vi "HTML Index Save.vi"(8 "error in (no error)":errorcluster, 10 "title":string) -> (0 "error out":errorcluster)   [LabVIEW 2014, in "lvprj2html.lvlib"]
uses:
  lvprj2html.lvlib
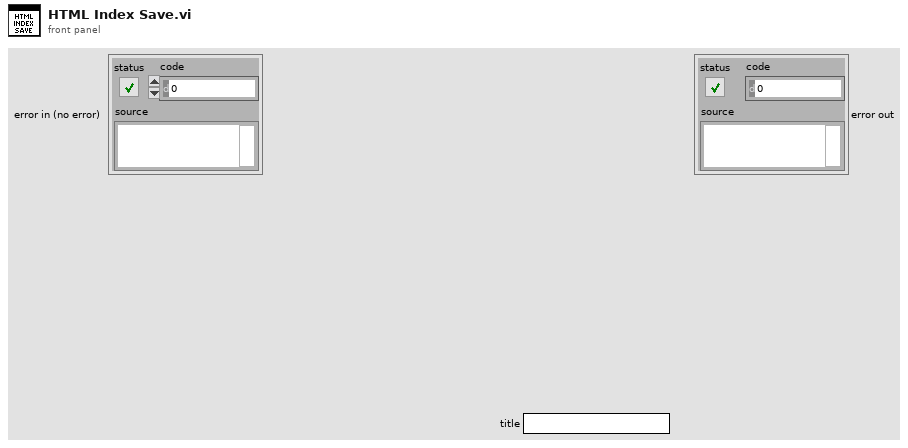
[diagram p1: front panel]
types:
  T1 = enum16{"open", "replace", "create", "open or create", "replace or create", "replace or create with confirmation"}
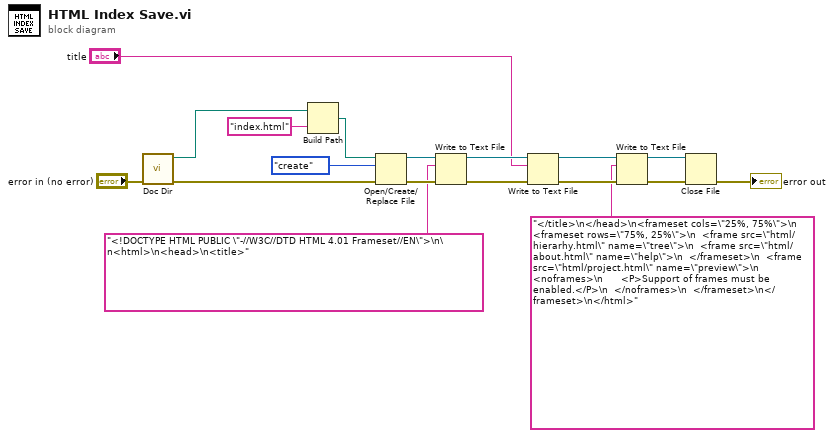
[diagram p0: block diagram]
diagram:
  n1 = call "Doc Dir.vi"("error in (no error)"="error in (no error)") -> ("error out"=w11:errorcluster, "appended path"=w12:path)  [unwired: 9 in]
  n2 = Build Path(base path=w12, name or relative path="index.html") -> (appended path=w16:path)
  n3 = Open/Create/Replace File(file path (use dialog)=w16, error in=w11, operation (0:open)=T1."create") -> (refnum out=w18:refnum<file>, error out=w14:errorcluster)  [unwired: 3 in, 1 out]
  n4 = Write to Text File(file (use dialog)=w18, text="<!DOCTYPE HTML PUBLIC \"-//W3C//DTD HTML 4.01 Frameset//EN\">\n\n<html>\n<head>\n<title>", error in=w14) -> (refnum out=w7:refnum<file>, error out=w4:errorcluster)  [unwired: 1 in, 1 out]
  n5 = Write to Text File(file (use dialog)=w7, text="title", error in=w4) -> (refnum out=w6:refnum<file>, error out=w5:errorcluster)  [unwired: 1 in, 1 out]
  n6 = Write to Text File(file (use dialog)=w6, text="</title>\n</head>\n<frameset cols=\"25%, 75%\">\n  <frameset rows=\"75%, 25%\">\n  <frame src=\"html/hierarhy.html\" name=\"tree\">\n  <frame src=\"html/about.html\" name=\"help\">\n  </frameset>\n  <frame src=\"html/project.html\" name=\"preview\">\n  <noframes>\n      <P>Support of frames must be enabled.</P>\n  </noframes>\n  </frameset>\n</frameset>\n</html>", error in=w5) -> (refnum out=w9:refnum<file>, error out=w10:errorcluster)  [unwired: 1 in, 1 out]
  n7 = Close File(refnum=w9, error in=w10) -> (error out=→"error out":errorcluster)  [unwired: 1 out]
